vi "Run.vi"(8 "error in (no error)":errorcluster, 11 "Terminal Timeout in":refnum<class "Terminal Timeout.lvclass">) -> (0 "error out":errorcluster, 3 "Terminal Timeout out":refnum<class "Terminal Timeout.lvclass">)   [LabVIEW 2016, in "CLD Exam - ATM.lvlib" / "Terminal Timeout.lvclass"]
uses:
  Terminal Timeout.lvclass
  D:/Repos/Stream/software/Mediator/Classes/Mediated Actor/Mediated Actor.lvclass
  Mediator/Classes/Message Interface/Message Interface.lvclass
  Terminal Timeout.lvclass/Terminal Timeout.ctl
  Mediator/Classes/Message String/Message String.lvclass
  D:/Repos/Stream/software/Mediator/Classes/Message Interface/Message Interface.lvclass
  Mediator/Classes/Message Transport Interface/Message Priority.ctl
  Log/Application Log/Log Level.ctl
  Mediator/Classes/Message Transport Queue/Message Transport Queue.lvclass
  D:/Repos/Stream/software/Mediator/Classes/Message Transport Interface/Message Transport Interface.lvclass
  Mediator/Classes/Mediated Actor/Mediated Actor.lvclass
  Mediator/Classes/Message Transport Interface/Message Transport Interface.lvclass
  Log/Application Log/Application Log.lvclass
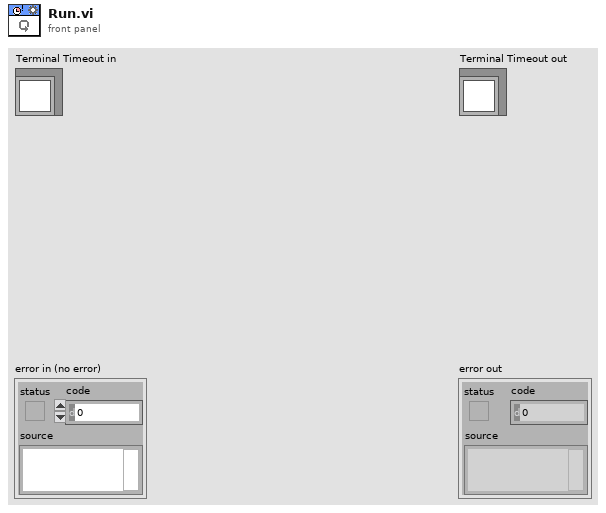
[diagram p1: front panel]
types:
  T1 = cluster{"Account Action Requested":refnum<event-registration>, "Card Inserted":refnum<event-registration>, "System Exit":refnum<event-registration>, "To Self":refnum<event-registration>}
  T2 = typedef "Stream Log.lvlib/Application Log.lvclass/Log Level.ctl" = enum16{"Imperative", "Major", "Minor", "Debug", "Off"}
  T3 = typedef "Stream Mediator.lvlib/Message Transport Interface.lvclass/Message Priority.ctl" = enum16{"Normal", "High"}
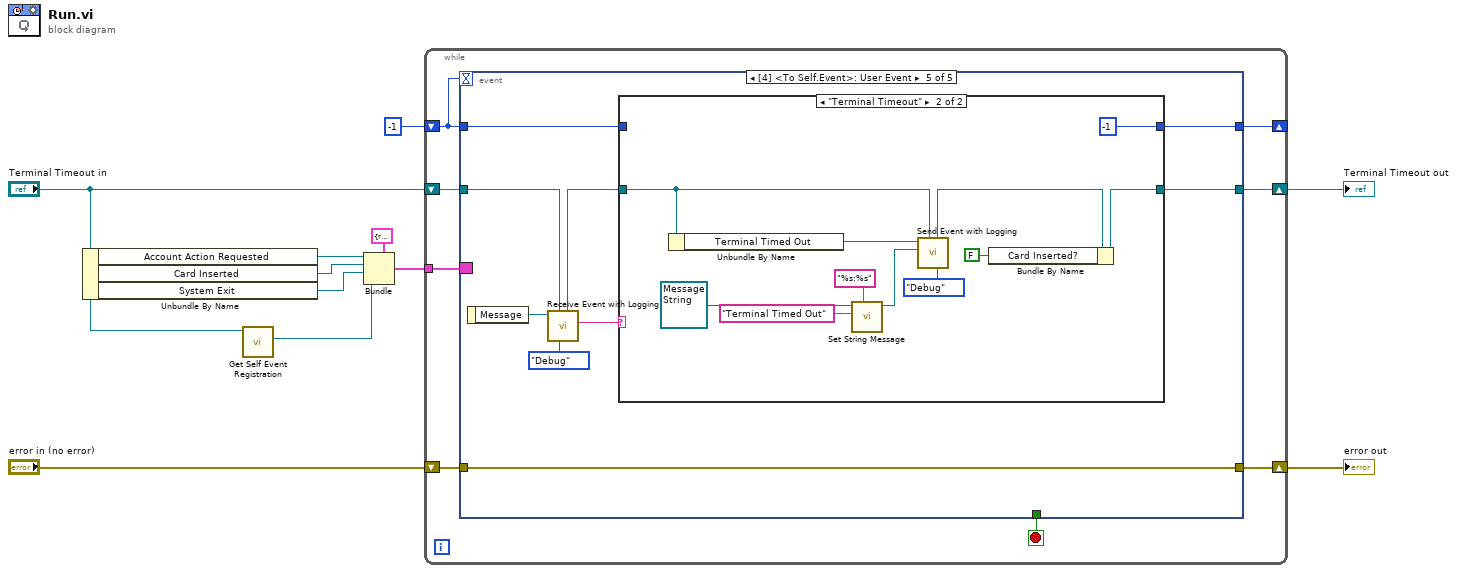
[diagram p0: block diagram]
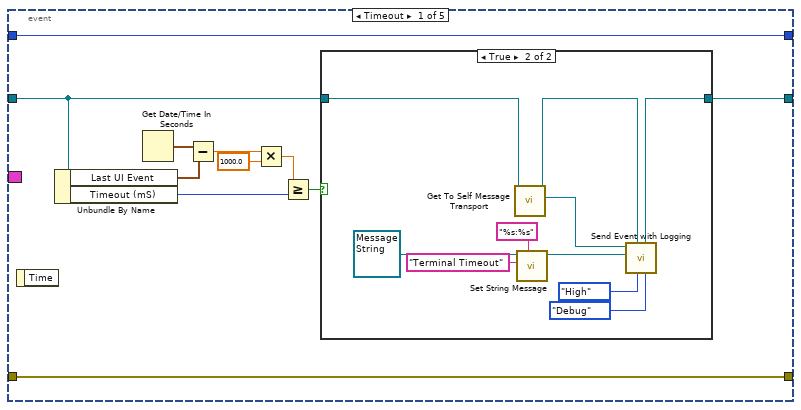
[diagram p2: hidden frame]
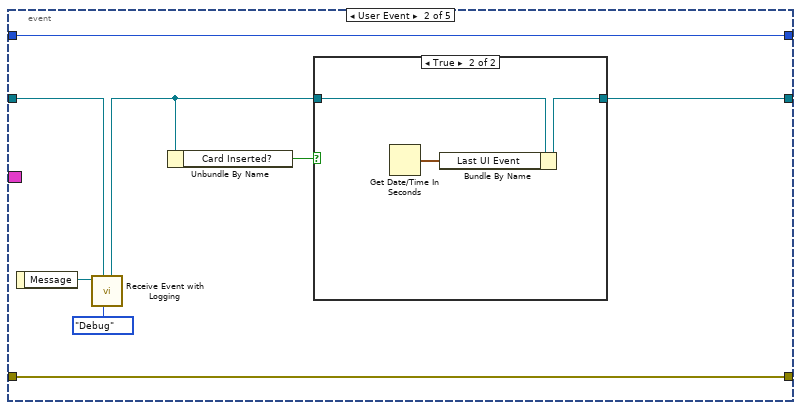
[diagram p4: hidden frame]
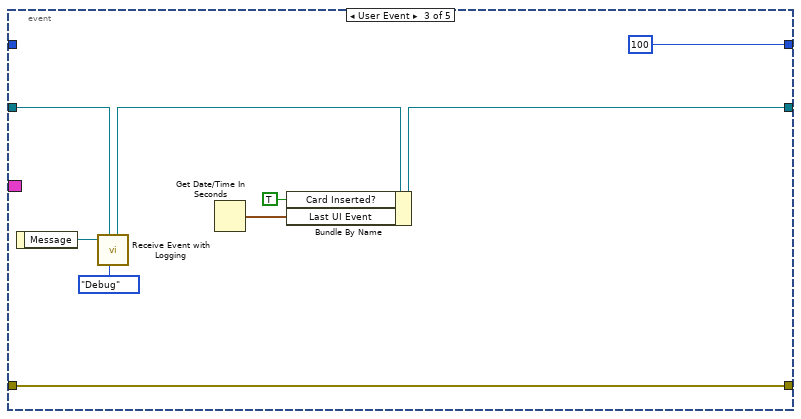
[diagram p6: hidden frame]
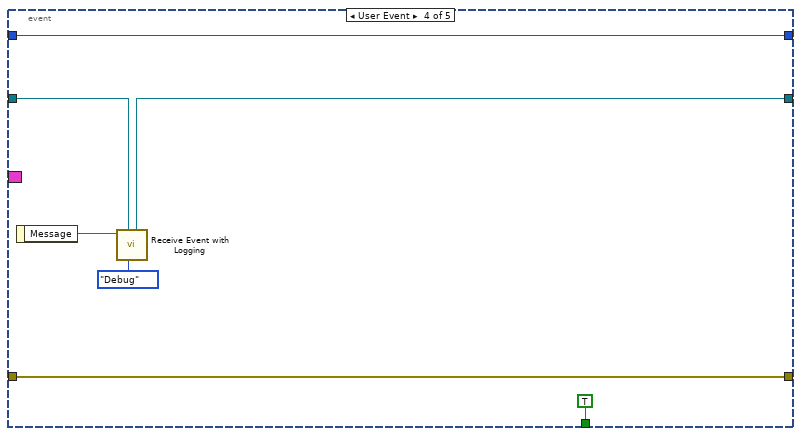
[diagram p7: hidden frame]
diagram:
  n1 = Unbundle By Name("Terminal Timeout in") -> ("Account Action Requested"=w10:refnum<event-registration>, "Card Inserted"=w9:refnum<event-registration>, "System Exit"=w8:refnum<event-registration>)
  n2 = call "Get Self Event Registration.vi"("Mediated Actor in"="Terminal Timeout in") -> ("Event Registration Refnum"=w6:refnum<event-registration>)  [unwired: 9 in, 1 out]
  n3 = Bundle(cluster=T1 {"Account Action Requested"=refnum, "Card Inserted"=refnum, "System Exit"=refnum, "To Self"=refnum}, "Account Action Requested"=w10, "Card Inserted"=w9, "System Exit"=w8, "To Self"=w6) -> (w2:T1)
  n4 = while {
    shift-right: [w18] -> w11
    shift-left: "Terminal Timeout in" -> [w19]
    tunnel: w2 -> [w17]
    shift-right: [w16] -> _
    shift-left: -1 -> [w15]
    shift-right: [w12] -> w3
    shift-left: "error in (no error)" -> [w13]
    stop <- w14 stop-if-true
    n5 = event shown="[4] <To Self.Event>: User Event" {
      selector: w17 -> [_ _ _ _ _]
      dyn-events: _ -> [_ _ _ _ _]
      timeout: w15 -> [_ _ _ _ _]
      tunnel: w19 -> [w23 w44 w55 w64 w71]
      tunnel: [w22 w47 w61 w63 w78] -> w18
      tunnel: w15 -> [w30 w49 _ w69 w77]
      tunnel: [w30 w49 100 w69 w76] -> w16
      tunnel: [_ _ _ TRUE _] -> w14
      tunnel: w13 -> [w20 w46 w58 w67 w75]
      tunnel: [w20 w46 w58 w67 w75] -> w12
      event Timeout {
        n6 = event-data() -> ()  [unwired: 1 in, 1 out]
        n7 = Unbundle By Name(w23) -> ("Last UI Event"=w28:timestamp, "Timeout (mS)"=w27:i32)
        n8 = Get Date/Time In Seconds() -> (seconds since 1Jan1904=w29:timestamp)
        n9 = Subtract(x=w29, y=w28) -> (x-y=w26:dbl)
        n10 = Multiply(x=w26, y=1000.0) -> (x*y=w25:dbl)
        n11 = Greater Or Equal?(x=w25, y=w27) -> (x >= y?=w21:bool)
        n12 = case shown="True" w21 {
          tunnel: w23 -> [w31 w39]
          tunnel: [w31 w34] -> w22
          frame False {
          }
          frame True {
            n13 = call "Get To Self Message Transport.vi"("Mediated Actor in"=w39) -> ("To Self"=w37:refnum<class "Message Transport Queue.lvclass">, "Mediated Actor out"=w35:refnum<class "Terminal Timeout.lvclass">)  [unwired: 9 in]
            n14 = call "Set String Message.vi"("Format"="%s:%s", "Name"="Terminal Timeout", "Message String in"=refnum<class "Message String.lvclass"> refnum) -> ("Message String out"=w36:refnum<class "Message String.lvclass">)  [unwired: 7 in, 1 out]
            n15 = call "Send Event with Logging.vi"("Global Log Level"=Log_Level."Debug", "Message Priority"=Message_Priority."High", "Mediated Actor in"=w35, "Message"=w36, "Message Transport Interface in"=w37) -> ("Mediated Actor out"=w34:refnum<class "Terminal Timeout.lvclass">)  [unwired: 5 in, 1 out]
          }
        }
      }
      event User Event {
        n16 = event-data() -> ("Message"=w45:refnum<class "Message Interface.lvclass">)  [unwired: 1 in]
        n17 = call "Receive Event with Logging.vi"("Global Log Level"=Log_Level."Debug", "Mediated Actor in"=w44, "Message"=w45) -> ("Mediated Actor out"=w43:refnum<class "Terminal Timeout.lvclass">)  [unwired: 5 in, 3 out]
        n18 = Unbundle By Name(w43) -> ("Card Inserted?"=w48:bool)
        n19 = case shown="True" w48 {
          tunnel: [w50 w52] -> w47
          tunnel: w43 -> [w50 w53]
          frame False {
          }
          frame True {
            n20 = Get Date/Time In Seconds() -> (seconds since 1Jan1904=w51:timestamp)
            n21 = Bundle By Name(cluster=w53, "Last UI Event"=w51) -> (w52:refnum<class "Terminal Timeout.lvclass">)
          }
        }
      }
      event User Event {
        n22 = event-data() -> ("Message"=w56:refnum<class "Message Interface.lvclass">)  [unwired: 1 in]
        n23 = call "Receive Event with Logging.vi"("Global Log Level"=Log_Level."Debug", "Mediated Actor in"=w55, "Message"=w56) -> ("Mediated Actor out"=w54:refnum<class "Terminal Timeout.lvclass">)  [unwired: 5 in, 3 out]
        n24 = Get Date/Time In Seconds() -> (seconds since 1Jan1904=w59:timestamp)
        n25 = Bundle By Name(cluster=w54, "Card Inserted?"=TRUE ("Data.Card Inserted?"), "Last UI Event"=w59) -> (w61:refnum<class "Terminal Timeout.lvclass">)
      }
      event User Event {
        n26 = event-data() -> ("Message"=w65:refnum<class "Message Interface.lvclass">)  [unwired: 1 in]
        n27 = call "Receive Event with Logging.vi"("Global Log Level"=Log_Level."Debug", "Mediated Actor in"=w64, "Message"=w65) -> ("Mediated Actor out"=w63:refnum<class "Terminal Timeout.lvclass">)  [unwired: 5 in, 3 out]
      }
      event User Event {
        n28 = event-data() -> ("Message"=w73:refnum<class "Message Interface.lvclass">)  [unwired: 1 in]
        n29 = call "Receive Event with Logging.vi"("Global Log Level"=Log_Level."Debug", "Mediated Actor in"=w71, "Message"=w73) -> ("Name"=w72:string, "Mediated Actor out"=w70:refnum<class "Terminal Timeout.lvclass">)  [unwired: 5 in, 2 out]
        n30 = case shown="\"Terminal Timeout\"" w72 {
          tunnel: [w80 w88] -> w78
          tunnel: w70 -> [w80 w83]
          tunnel: [w79 -1] -> w76
          tunnel: w77 -> [w79 _]
          frame Default {
          }
          frame "Terminal Timeout" {
            n31 = Unbundle By Name(w83) -> ("Terminal Timed Out"=w85:refnum<class "Message Transport Queue.lvclass">)
            n32 = call "Set String Message.vi"("Format"="%s:%s", "Name"="Terminal Timed Out", "Message String in"=refnum<class "Message String.lvclass"> refnum) -> ("Message String out"=w84:refnum<class "Message String.lvclass">)  [unwired: 7 in, 1 out]
            n33 = call "Send Event with Logging.vi"("Global Log Level"=Log_Level."Debug", "Mediated Actor in"=w83, "Message"=w84, "Message Transport Interface in"=w85) -> ("Mediated Actor out"=w82:refnum<class "Terminal Timeout.lvclass">)  [unwired: 6 in, 1 out]
            n34 = Bundle By Name(cluster=w82, "Card Inserted?"=FALSE ("Data.Card Inserted?")) -> (w88:refnum<class "Terminal Timeout.lvclass">)
          }
        }
      }
    }
  }
  "error out" <- w3
  "Terminal Timeout out" <- w11
